vi "control-shutter-subvi.vi"(8 "Error In":errorcluster, 11 "Shutter Control":T1) -> (0 "Error Out":errorcluster)   [LabVIEW 2014]
uses:
  ctts/user event shutter global.ctl
  Global Shutter Variables - SubVI.vi
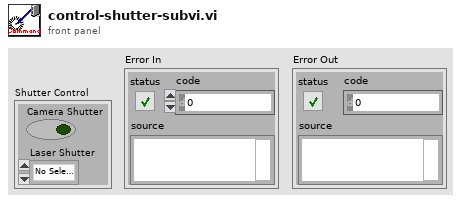
[diagram p1: front panel]
types:
  T1 = typedef "user event shutter global.ctl" = cluster{"Camera Shutter":bool, "Laser Shutter":enum32{"No Selection", "GFP", "Cy3 Long \nPass", "Cy3", "Cy5", "Off", "IR"}}
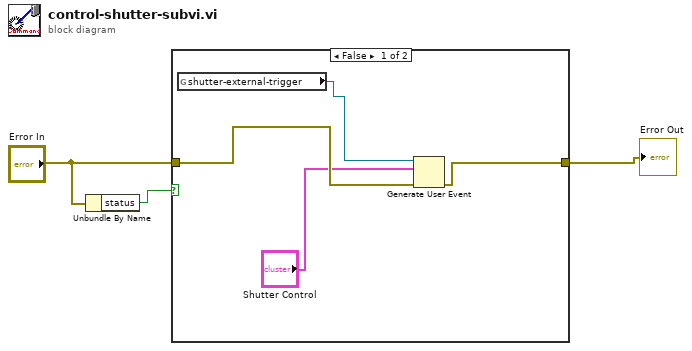
[diagram p0: block diagram]
diagram:
  n1 = Unbundle By Name("Error In") -> ("status"=w2:bool)
  n2 = case shown="False" w2 {
    tunnel: [w7 w8] -> w3
    tunnel: "Error In" -> [w6 w8]
    frame False {
      n3 = global read "Global Shutter Variables - SubVI.vi" "shutter-external-trigger"() -> (w4:refnum<user-event>)
      n4 = Generate User Event(user event=w4, event data cluster="Shutter Control", error in=w6) -> (error out=w7:errorcluster)  [unwired: 1 in, 1 out]
    }
    frame True {
    }
  }
  "Error Out" <- w3
